vi "Newmark-Stop.vi"(0 "Table VRN IN":refnum<visa-resource-name>="COM9", 2 "Bool Refnum":refnum<vi>, 11 "Error IN":errorcluster) -> (4 "Table VRN OUT":refnum<visa-resource-name>="COM9", 15 "Error OUT":errorcluster)   [LabVIEW 2019]
uses:
  Comm/SerialCommError.vi
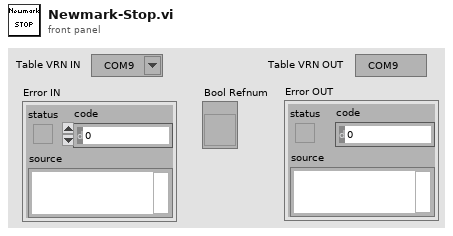
[diagram p1: front panel]
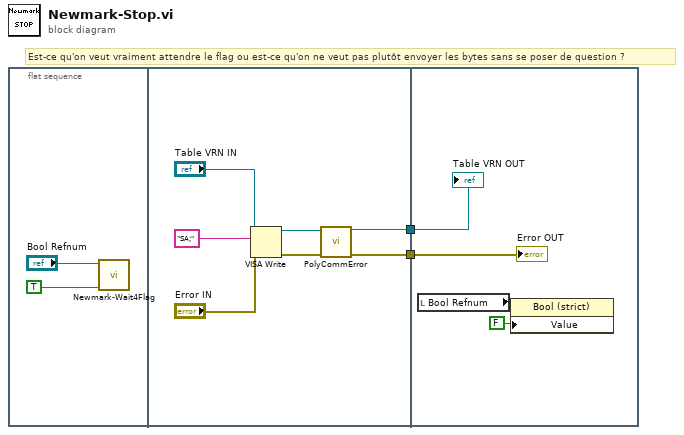
[diagram p0: block diagram]
diagram:
  # "Est-ce qu'on veut vraiment attendre le flag ou est-ce qu'on ne veut pas plutôt envoyer les bytes sans se poser de question ?"
  n1 = flat-sequence {
    tunnel: [w6] -> w2
    tunnel: [w5] -> w1
    tunnel: w2 -> [w15]
    tunnel: w1 -> [w14]
    frame #0 {
      n2 = call "Newmark-Wait4Flag.vi"("Raise Flag ?"=TRUE, "Ctl Refnum IN"="Bool Refnum") -> ()  [unwired: 8 in, 2 out]
    }
    frame #1 {
      n3 = VISA Write(VISA resource name="Table VRN IN", write buffer="SA;", error in (no error)="Error IN") -> (VISA resource name out=w8:refnum<visa-resource-name>, error out=w7:errorcluster)  [unwired: 1 out]
      n4 = call-poly "PolyCommError.vi"("VISA IN"=w8, "error IN"=w7) -> ("VISA OUT"=w6:refnum<visa-resource-name>, "error OUT"=w5:errorcluster)  [unwired: 11 in, 1 out]
    }
    frame #2 {
      n5 = local read "Bool Refnum"() -> (w13:refnum<vi>)
      n6 = property class="Bool (strict)"(reference=w13, "Value"=FALSE) -> ()  [unwired: 1 in, 2 out]
      "Error OUT" <- w14
      "Table VRN OUT" <- w15
    }
  }
